vi "CellValueChanged Event Callback.vi"(4 "DataGridView in":refnum<class "DataGridView.lvclass">, 5 "Event Data":cluster{"sender":refnum<k24>, "e":refnum<k24>}, 6 "Control Ref":refnum<k24>, 7 "Event Common Data":T1) -> ()   [LabVIEW 2013, in "DataGrid.lvlib" / "DataGridView.lvclass"]
uses:
  DataGridView/DataGridView.lvclass
  System.Windows.Forms
  CellValueChanged/CellValueChanged.lvclass
  CellValueChanged/CellValueChanged.lvclass/CellValueChanged.ctl
  CellValueChanged/Write cell value.vi
  CellValueChanged/Write row.vi
  CellValueChanged/Write column.vi
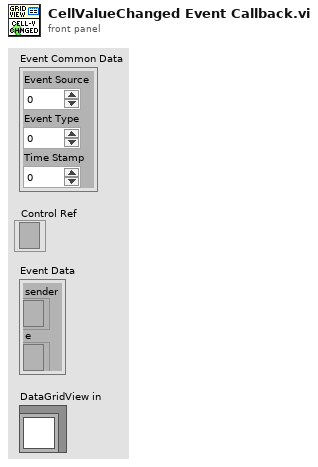
[diagram p1: front panel]
types:
  T1 = cluster{"Event Source":i32, "Event Type":u32, "Time Stamp":u32}
  T2 = cluster{"CellClicked":refnum<user-event>, "CellValue Changed":refnum<user-event>, "KeyDown":refnum<user-event>, "DataError":refnum<user-event>, "UserAddedRow":refnum<user-event>, "UserDeletedRow":refnum<user-event>}
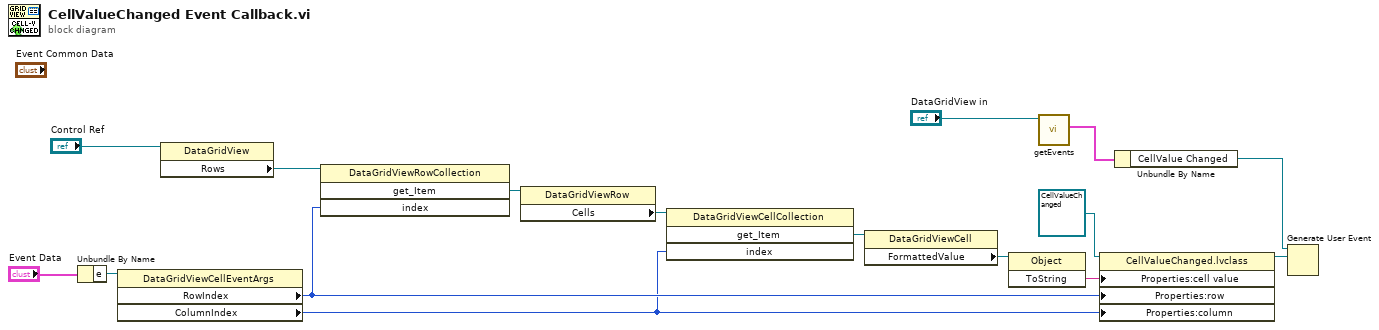
[diagram p0: block diagram]
diagram:
  n1 = Unbundle By Name("Event Data") -> ("e"=w12:refnum<k24>)
  n2 = property class="DataGridViewCellEventArgs"(reference=w12) -> ("RowIndex"=w8:i32, "ColumnIndex"=w5:i32)  [unwired: 1 in, 2 out]
  n3 = property class="DataGridView"(reference="Control Ref") -> ("Rows"=w9:refnum<k24>)  [unwired: 1 in, 2 out]
  n4 = invoke class="DataGridViewRowCollection" method="get_Item"(reference=w9, "index"=w8) -> ("get_Item"=w7:refnum<k24>)  [unwired: 2 in, 3 out]
  n5 = property class="DataGridViewRow"(reference=w7) -> ("Cells"=w6:refnum<k24>)  [unwired: 1 in, 2 out]
  n6 = invoke class="DataGridViewCellCollection" method="get_Item"(reference=w6, "index"=w5) -> ("get_Item"=w4:refnum<k24>)  [unwired: 2 in, 3 out]
  n7 = property class="DataGridViewCell"(reference=w4) -> ("FormattedValue"=w3:refnum<k24>)  [unwired: 1 in, 2 out]
  n8 = invoke class="Object" method="ToString"(reference=w3) -> ("ToString"=w2:string)  [unwired: 2 in, 2 out]
  n9 = call "getEvents.vi"("DataGridView in"="DataGridView in") -> ("userEvents"=w16:T2)  [unwired: 8 in, 2 out]
  n10 = property class="CellValueChanged.lvclass"(reference=refnum<class "CellValueChanged.lvclass"> refnum ("DataGrid.lvlib:CellValueChanged.lvclass"), "Properties:cell value"=w2, "Properties:row"=w8, "Properties:column"=w5) -> (reference out=w1:refnum<class "CellValueChanged.lvclass">)  [unwired: 1 in, 1 out]
  n11 = Unbundle By Name(w16) -> ("CellValue Changed"=w15:refnum<user-event>)
  n12 = Generate User Event(user event=w15, event data cluster=w1) -> ()  [unwired: 2 in, 2 out]
